vi "Write Statement_id.vi"(10 "Statement_id":i32, 11 "Result in":refnum<class "Result.lvclass">) -> (3 "Result out":refnum<class "Result.lvclass">)   [LabVIEW 2018, in "InfluxDB Client.lvlib" / "Result.lvclass"]
uses:
  Result.lvclass
  Result.lvclass/Result.ctl
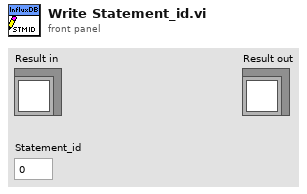
[diagram p1: front panel]
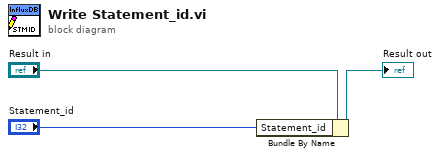
[diagram p0: block diagram]
diagram:
  n1 = Bundle By Name(cluster="Result in", "Statement_id"="Statement_id") -> (→"Result out":refnum<class "Result.lvclass">)
